vi "Mask Byte Array To Bit Array.vi"(9 "Height":i16, 10 "Width":i16, 11 "Mask Byte Array":u8[](array[numeric])) -> (3 "Mask Bit Array":bool[](array[boolean]))   [LabVIEW 2020, in "G-Image.lvlib"]
uses:
  G-Image.lvlib
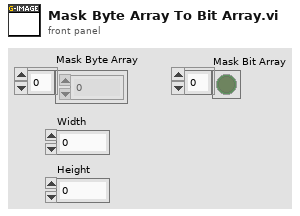
[diagram p1: front panel]
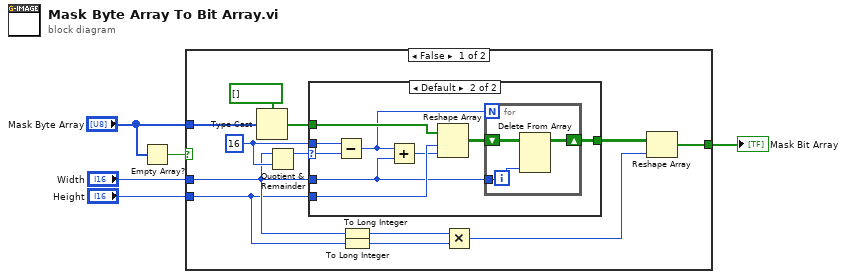
[diagram p0: block diagram]
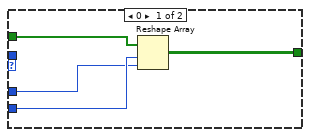
[diagram p2: hidden frame]
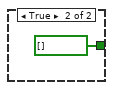
[diagram p3: hidden frame]
diagram:
  n1 = Empty Array?(array="Mask Byte Array") -> (empty?=w2:bool)
  n2 = case shown="False" w2 {
    tunnel: "Mask Byte Array" -> [w12 _]
    tunnel: "Width" -> [w10 _]
    tunnel: "Height" -> [w9 _]
    tunnel: [w8 bool[] []] -> w1
    frame False {
      w13 = i16 16 ("y")
      n3 = Type Cast(type=bool[] [], x=w12) -> (*(type *) &x=w16:bool[])
      n4 = Quotient & Remainder(x=w10, y=w13) -> (x-y*floor(x/y)=w14:i16)  [unwired: 1 out]
      n5 = case shown="Default" w14 {
        selector: w14 -> [_ w23]
        tunnel: w16 -> [w21 w30]
        tunnel: [w18 w28] -> w15
        tunnel: w9 -> [w20 w27]
        tunnel: w10 -> [w19 w26]
        tunnel: w13 -> [_ w24]
        frame 0 {
          n6 = Reshape Array(w21, w20, w19) -> (w18:bool[][])
        }
        frame Default {
          n7 = Subtract(x=w24, y=w23) -> (x-y=w22:i16)
          n8 = Add(x=w22, y=w26) -> (x+y=w25:i16)
          n9 = Reshape Array(w30, w27, w25) -> (w29:bool[][])
          n10 = for {
            N: w22 -> [_]
            shift-right: [w32] -> w28
            shift-left: w29 -> [w33]
            tunnel: w26 -> [w31]
            n11 = Delete From Array(array=w33, index (col)=w31) -> (array with subset deleted=w32:bool[][])  [unwired: 2 in, 1 out]
          }
        }
      }
      n12 = To Long Integer(number=w10) -> (32bit integer=w7:i32)
      n13 = To Long Integer(number=w9) -> (32bit integer=w6:i32)
      n14 = Multiply(x=w7, y=w6) -> (x*y=w11:i32)
      n15 = Reshape Array(w15, w11) -> (w8:bool[])
    }
    frame True {
    }
  }
  "Mask Bit Array" <- w1
